vi "Initialize Session.vi"(8 "error in":errorcluster, 10 "Port":refnum<visa-resource-name>="COM13", 11 "Airmar WS in":refnum<class "Airmar WS.lvclass">) -> (0 "error out":errorcluster, 3 "Airmar WS out":refnum<class "Airmar WS.lvclass">)   [LabVIEW 2014, in "Airmar WS.lvclass"]
uses:
  Airmar WS.lvclass
  Airmar WS.lvclass/Airmar WS.ctl
  Reusable/Session APIs/Serial/Serial Session.lvclass
  <userlib>/_Session Fwk/Session - Root.lvclass
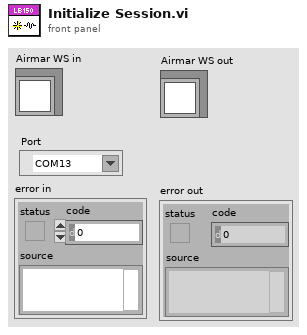
[diagram p1: front panel]
types:
  T1 = cluster{"baud rate (9600)":u32, "data bits (8)":u16, "stop bits (10: 1 bit)":u16, "parity (0:none)":enum16{"None", "Odd", "Even", "Mark", "Space"}, "flow control (0:none)":u16, "endModeforReads":u16, "endModeforWrites":u16}
  T2 = cluster{"EnTermChar":bool, "termChar":u8, "suppEnEnRd":bool, "sendEndEn":bool}
  T3 = typedef "Session - Root.lvclass/Session Handle.ctl" = refnum<data-value>
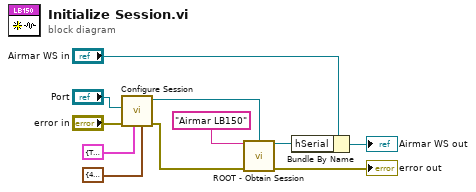
[diagram p0: block diagram]
diagram:
  n1 = call "Configure Session.vi"("serialCfg"=T1 {"baud rate (9600)"=4800, "data bits (8)"=8, "stop bits (10: 1 bit)"=10, "parity (0:none)"=enum."None", "flow control (0:none)"=0, "endModeforReads"=2, "endModeforWrites"=2}, "Message Cfg"=T2 {"EnTermChar"=TRUE, "termChar"=10, "suppEnEnRd"=FALSE, "sendEndEn"=TRUE} ("Message Cfg 2"), "error in"="error in", "VISA Resource"="Port") -> ("error out"=w2:errorcluster, "Serial Session out"=w5:refnum<class "Serial Session.lvclass">)  [unwired: 6 in]
  n2 = call <userlib>:"ROOT - Obtain Session.vi"("Session Name ()"="Airmar LB150", "OBJ - Session"=w5, "error in (no error)"=w2) -> ("Session Handle"=w4:T3, "error out"=→"error out":errorcluster)  [unwired: 10 in, 1 out]
  n3 = Bundle By Name(cluster="Airmar WS in", "hSerial"=w4) -> (→"Airmar WS out":refnum<class "Airmar WS.lvclass">)
